vi "move V1.2.vi"(8 "error in (no error)":errorcluster, 9 "RPM":dbl, 10 "Y":dbl, 11 "X":dbl) -> (0 "error out":errorcluster)   [LabVIEW 2019]
uses:
  <vilib>/Platform/TimedLoop/XDataNode/timing_clust.ctl
  <vilib>/Platform/TimedLoop/XDataNode/nitl_modes.ctl
  <vilib>/Platform/TimedLoop/XDataNode/wakeup.ctl
  <vilib>/addons/control/pid/pid.llb/PID (DBL).vi
  <vilib>/platform/TimedLoop/XDataNode/XDataNode.xnode
  <vilib>/Platform/TimedLoop/XDataNode/XDNodeRunTimeDep.lvlib
  <vilib>/addons/control/pid/NI_PID_pid.lvlib
panel:
  out "AC estimate (Vrms)":dbl format="%0.2f"
  out "out array":dbl[](array[numeric])
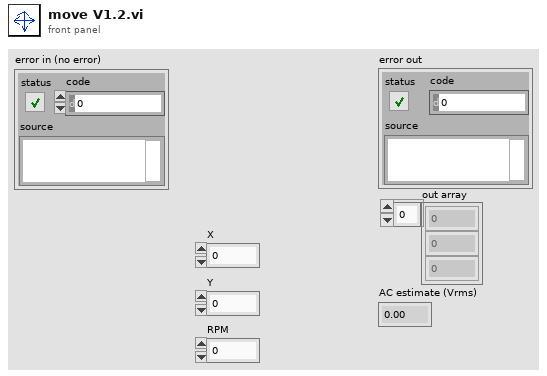
[diagram p1: front panel]
types:
  T1 = typedef "XDNodeRunTimeDep.lvlib/timing_clust.ctl" = cluster{"Expected End [f-1]":u64, "Actual End [f-1]":u64, "Finished Late? [f-1]":bool, "Expected End [i-1]":u64, "Actual End [i-1]":u64, "Finished Late? [i-1]":bool, "Expected Start [i]":u64, "Actual Start [i]":u64, "Expected Start [f]":u64, "Actual Start [f]":u64, "Source Name":string, "Structure Name":string, "Period":i64, "Deadline":i64, "Offset":i64, "Start":i64, "Priority":i32, "Timeout":i32, "Mode":T2, "Wakeup Reason":T3, "Error":errorcluster, "Source Type":string, "Secondary Source Type":string, "Global End Time":u64, "Global Start Time":u64, "Frame Duration":u64, "Iteration Duration":u64, "Assigned CPU":i32, "I/O Scan Engine Mode":u32}
  T2 = typedef "XDNodeRunTimeDep.lvlib/nitl_modes.ctl" = enum32{"No Change", "Process missed periods, maintain original phase", "Discard missed periods, maintain original phase", "Process missed periods, ignore original phase", "Discard missed periods, ignore original phase"}
  T3 = typedef "XDNodeRunTimeDep.lvlib/wakeup.ctl" = enum32{"Normal", "Aborted", "Asynchronous wakeup", "Timing source error", "Timed loop error", "Timeout"}
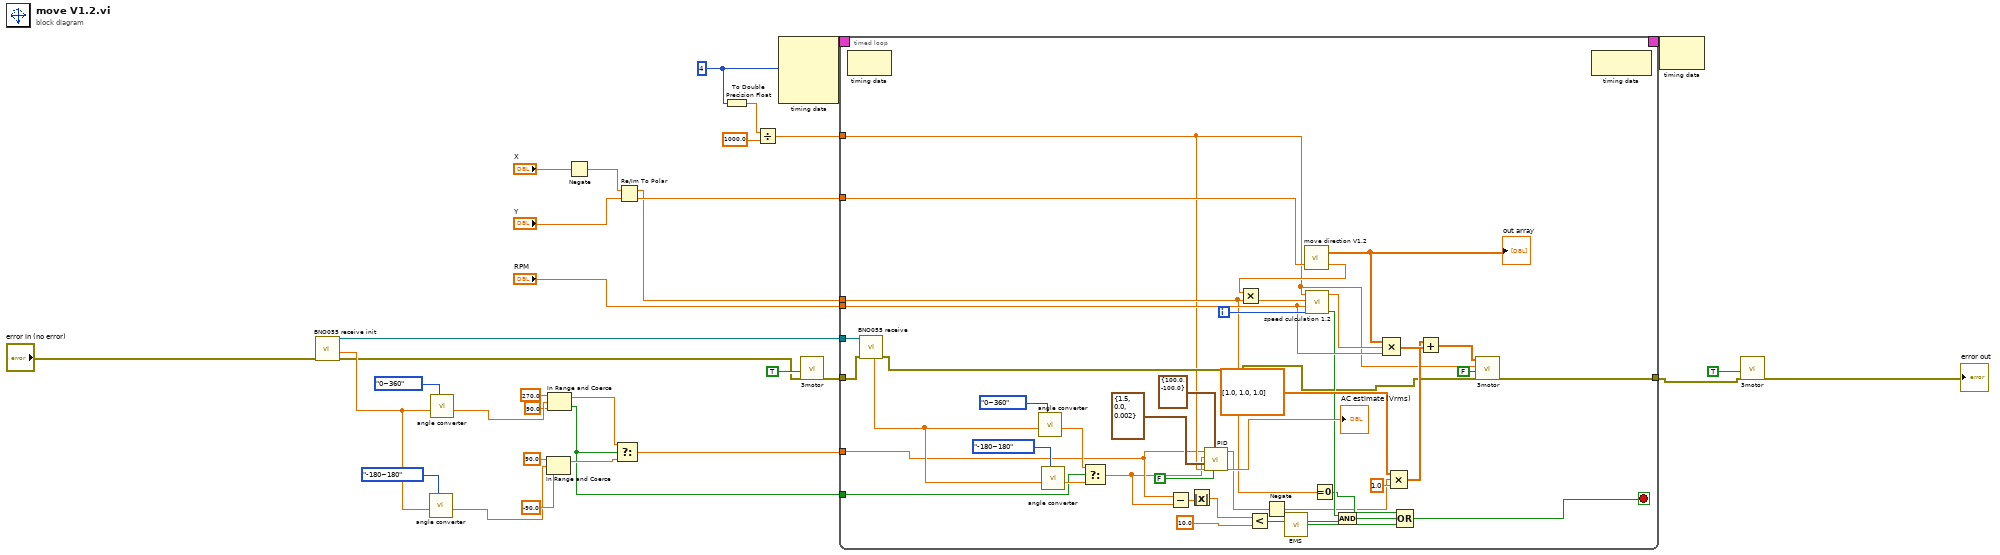
[diagram p0: block diagram]
diagram:
  w31 = i64 4 ("Period")
  n1 = call "BNO055 receive init.vi"("error in (no error)"="error in (no error)") -> ("error out"=w5:errorcluster, "element"=w9:dbl, "rt fifo out"=w3:refnum<k33>)  [unwired: 8 in]
  n2 = call "angle converter.vi"("select"=enum16{"-180~180", "0~360"}."-180~180", "input angle"=w9) -> ("angle out"=w17:dbl)  [unwired: 9 in]
  n3 = call "angle converter.vi"("select"=enum16{"-180~180", "0~360"}."0~360", "input angle"=w9) -> ("angle out"=w14:dbl)  [unwired: 9 in]
  n4 = In Range and Coerce(upper limit=90.0, x=w17, lower limit=-90.0) -> (coerced(x)=w10:dbl)  [unwired: 1 out]
  n5 = In Range and Coerce(upper limit=270.0, x=w14, lower limit=90.0) -> (coerced(x)=w11:dbl, In Range?=w7:bool)
  n6 = Negate(x="X") -> (-x=w4:dbl)
  n7 = Select(t=w11, s=w7, f=w10) -> (s? t:f=w8:dbl)
  n8 = Re/Im To Polar(2:"Y", 3:w4) -> (0:w26:dbl, 1:w25:dbl)
  n9 = To Double Precision Float(number=w31) -> (double precision float=w30:dbl)
  n10 = Divide(x=w30, y=1000.0) -> (x/y=w28:dbl)
  n11 = node-c288(w31) -> (w33:T1)  [unwired: 3 in]
  n12 = call "3motor.vi"("error in (no error)"=w5, "Reset"=TRUE) -> ("error out"=w23:errorcluster)  [unwired: 8 in, 1 out]
  n13 = timed-loop {
    timing: w33 -> [_]
    timing-out: [_] -> w32
    tunnel: w28 -> [w46]
    tunnel: w26 -> [w74]
    tunnel: w25 -> [w51]
    tunnel: "RPM" -> [w65]
    tunnel: w23 -> [w48]
    tunnel: [w72] -> w2
    tunnel: w8 -> [w41]
    tunnel: w7 -> [w59]
    tunnel: w3 -> [w50]
    i -> [w75]
    stop <- w53 stop-if-true
    n14 = node-c288() -> ()  [unwired: 1 in, 1 out]
    n15 = call "BNO055 receive.vi"("error in (no error)"=w48, "rt fifo"=w50) -> ("error out"=w49:errorcluster, "out"=w44:dbl)  [unwired: 7 in, 1 out]
    n16 = call "angle converter.vi"("select"=enum16{"-180~180", "0~360"}."0~360", "input angle"=w44) -> ("angle out"=w61:dbl)  [unwired: 9 in]
    n17 = call "angle converter.vi"("select"=enum16{"-180~180", "0~360"}."-180~180", "input angle"=w44) -> ("angle out"=w60:dbl)  [unwired: 9 in]
    n18 = Select(t=w61, s=w59, f=w60) -> (s? t:f=w40:dbl)
    n19 = Subtract(x=w41, y=w40) -> (x-y=w39:dbl)
    n20 = Absolute Value(x=w39) -> (abs(x)=w38:dbl)
    n21 = call-poly <vilib>:"PID.vi"("reinitialize? (F)"=FALSE, "output range"=cluster{"output high":dbl, "output low":dbl} {"output high"=100.0, "output low"=-100.0}, "dt (s)"=w46, "PID gains"=cluster{"Kp":dbl, "Ki":dbl, "Kd":dbl} {"Kp"=1.5, "Ki"=0.0, "Kd"=0.002} ("PID"), "process variable"=w40, "setpoint"=w41) -> ("dt out (s)"=→"AC estimate (Vrms)":dbl, "output"=w45:dbl)  [unwired: 4 in]
    n22 = Less?(x=w38, y=10.0) -> (x < y?=w36:bool)
    n23 = Negate(x=w45) -> (-x=w34:dbl)
    n24 = call "EMS.vi"() -> ("A/DIO4 (Pin 19)"=w47:bool)
    n25 = call "move direction V1.2.vi"("theta"=w74) -> ("max value"=w66:dbl, "out array"=w73:dbl[])  [unwired: 1 in]
    "out array" <- w73
    n26 = Multiply(x=w66, y=w51) -> (x*y=w67:dbl)
    n27 = call "speed culculation 1.2.vi"("i"=w75, "Speed(RPM)"=w65, "distance"=w67, "dt(s)"=w46) -> ("complet?"=w54:bool, "Speed"=w69:dbl)  [unwired: 4 in, 2 out]
    n28 = Equal To 0?(x=w51) -> (x = 0?=w52:bool)
    n29 = And(x=w54, y=w36) -> (x .and. y?=w42:bool)
    n30 = Compound Arithmetic op=MULTIPLY(w73, w69, w65) -> (w71:dbl[])
    n31 = Compound Arithmetic op=MULTIPLY(dbl[] [1.0, 1.0, 1.0], w34, 1.0 ("value")) -> (w70:dbl[])
    n32 = Compound Arithmetic op=OR(w52, w42, w47) -> (w53:bool)
    n33 = Add(x=w70, y=w71) -> (x+y=w68:dbl[])
    n34 = call "3motor.vi"("error in (no error)"=w49, "Reset"=FALSE, "dt(s)"=w46, "Motor speed"=w68) -> ("error out"=w72:errorcluster)  [unwired: 6 in, 1 out]
    n35 = node-c288() -> ()  [unwired: 1 in, 1 out]
  }
  n36 = node-c288(w32) -> ()  [unwired: 1 out]
  n37 = call "3motor.vi"("error in (no error)"=w2, "Reset"=TRUE) -> ("error out"=→"error out":errorcluster)  [unwired: 8 in, 1 out]
